vi "MaxLines.vi"(8 "error in (no error)":errorcluster, 10 "Camera Settings":T1={"Exposure Time (ms)"=100.0, "Binning"=enum."2x2", "Scan Mode"=0, "Frames to Acquire"=1000.0, "Pixel Correction"=FALSE, "Frames to Skip"=0, "File Path"=path "", "Duty cycle"=0.0, "ALEX"=FALSE, "Shutter Enable"=[], "fluidics trigger frame"=0, "Bit Depth"=0, "Image Width (px)"=0, "Image Height (px)"=0, "Horizontal Offset (px)"=0, "Vertical Offset (px)"=0} {"fluidics trigger frame" max=60000 step=1; "Exposure Time (ms)" min=1.0 max=10000.0 step=1.0}, 11 "Andor Camera in":refnum<class "Andor Camera.lvclass">) -> (0 "error out":errorcluster, 2 "Camera Settings 2":T1={"Exposure Time (ms)"=100.0, "Binning"=enum."2x2", "Scan Mode"=0, "Frames to Acquire"=1000.0, "Pixel Correction"=FALSE, "Frames to Skip"=0, "File Path"=path "", "Duty cycle"=0.0, "ALEX"=FALSE, "Shutter Enable"=[], "fluidics trigger frame"=0, "Bit Depth"=0, "Image Width (px)"=0, "Image Height (px)"=0, "Horizontal Offset (px)"=0, "Vertical Offset (px)"=0} {"fluidics trigger frame" max=60000 step=1; "Exposure Time (ms)" min=1.0 max=10000.0 step=1.0}, 3 "Andor Camera out":refnum<class "Andor Camera.lvclass">)   [LabVIEW 2018, in "Andor Camera.lvlib" / "Andor Camera.lvclass"]
uses:
  Andor Camera.lvclass
  Resources/Type Defs/Camera Settings.ctl
  Andor Camera.lvclass/Andor Camera.ctl
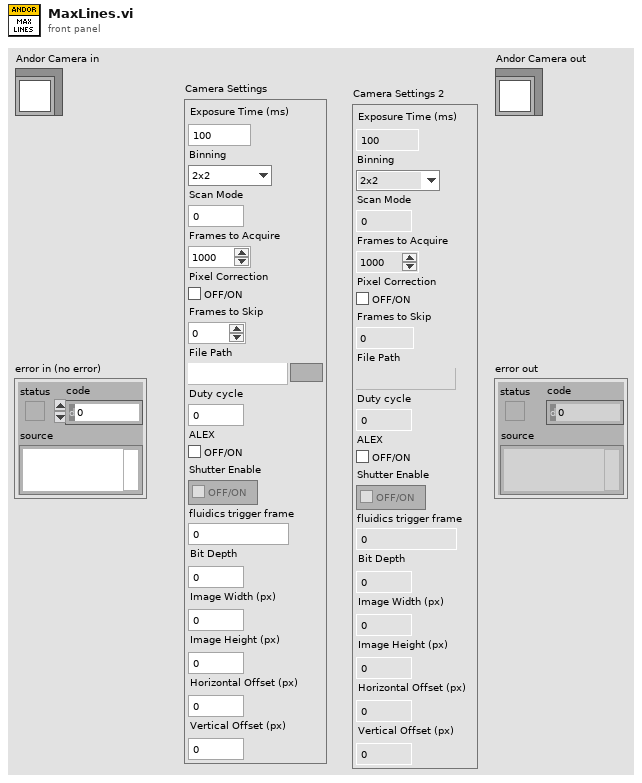
[diagram p1: front panel]
types:
  T1 = typedef "Camera Settings.ctl" = cluster{"Exposure Time (ms)":dbl, "Binning":enum16{"1x1", "2x2", "4x4"}, "Scan Mode":i32, "Frames to Acquire":dbl, "Pixel Correction":bool, "Frames to Skip":u32, "File Path":path, "Duty cycle":dbl, "ALEX":bool, "Shutter Enable":bool[], "fluidics trigger frame":u16, "Bit Depth":u16, "Image Width (px)":u16, "Image Height (px)":u16, "Horizontal Offset (px)":u16, "Vertical Offset (px)":u16}
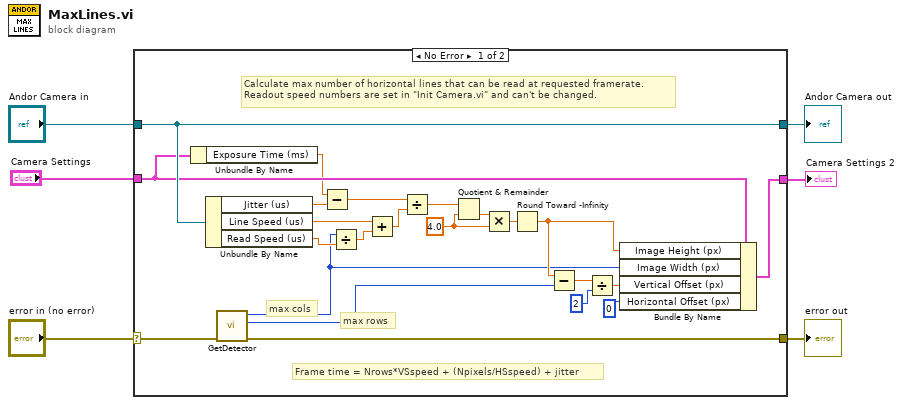
[diagram p0: block diagram]
diagram:
  n1 = case shown="No Error" "error in (no error)" {
    selector: "error in (no error)" -> [w28 w32]
    tunnel: [w27 w32] -> w5
    tunnel: [w23 w31] -> w3
    tunnel: "Andor Camera in" -> [w23 w31]
    tunnel: "Camera Settings" -> [w22 w30]
    tunnel: [w29 w30] -> w1
    frame No Error {
      w12 = 4.0 ("y")
      # "max cols"
      # "max rows"
      # "Frame time = Nrows*VSspeed + (Npixels/HSspeed) + jitter"
      # "Calculate max number of horizontal lines that can be read at requested framerate.\nReadout speed numbers are set in \"Init Camera.vi\" and can't be changed."
      n2 = Unbundle By Name(w22) -> ("Exposure Time (ms)"=w21:dbl)
      n3 = Unbundle By Name(w23) -> ("Jitter (us)"=w20:dbl, "Line Speed (us)"=w19:dbl, "Read Speed (us)"=w18:dbl)
      n4 = call <userlib>:"GetDetector.vi"("error in (no error)"=w28) -> ("error out"=w27:errorcluster, "ypixels"=w9:i32, "xpixels"=w7:i32)  [unwired: 3 in, 1 out]
      n5 = Subtract(x=w21, y=w20) -> (x-y=w16:dbl)
      n6 = Divide(x=w7, y=w18) -> (x/y=w17:dbl)
      n7 = Add(x=w19, y=w17) -> (x+y=w15:dbl)
      n8 = Divide(x=w16, y=w15) -> (x/y=w14:dbl)
      n9 = Quotient & Remainder(x=w14, y=w12) -> (floor(x/y)=w13:dbl)  [unwired: 1 out]
      n10 = Multiply(x=w13, y=w12) -> (x*y=w11:dbl)
      n11 = Round Toward -Infinity(1:w11) -> (0:w8:dbl)
      n12 = Subtract(x=w8, y=w9) -> (x-y=w25:dbl)
      n13 = Divide(x=w25, y=2) -> (x/y=w26:dbl)
      n14 = Bundle By Name(cluster=w22, "Image Height (px)"=w8, "Image Width (px)"=w7, "Vertical Offset (px)"=w26, "Horizontal Offset (px)"=u16 0) -> (w29:T1)
    }
    frame Error {
    }
  }
  "error out" <- w5
  "Andor Camera out" <- w3
  "Camera Settings 2" <- w1
